vi "Read Array of the pixel to zone correspondences.vi"(8 "error in (no error)":errorcluster, 11 "Data in":refnum<class "Data.lvclass">) -> (0 "error out":errorcluster, 2 "Pixel <> Zone":T1, 3 "Data out":refnum<class "Data.lvclass">)   [LabVIEW 2018, in "Data.lvclass"]
uses:
  Data.lvclass
  SubVi's/Controls/CTL_Pixel_to_Zone_array.ctl
  Data.lvclass/Data.ctl
  Common_Resources.lvlib
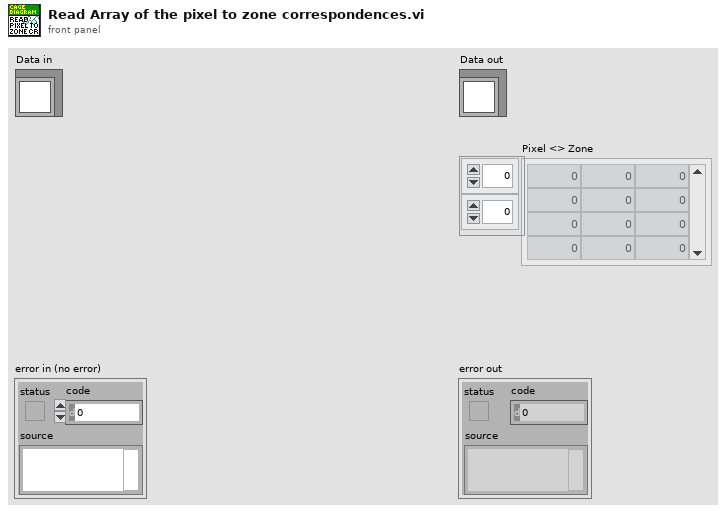
[diagram p1: front panel]
types:
  T1 = typedef "Common_Resources.lvlib/CTL_Pixel_to_Zone_array.ctl" = i8[][]
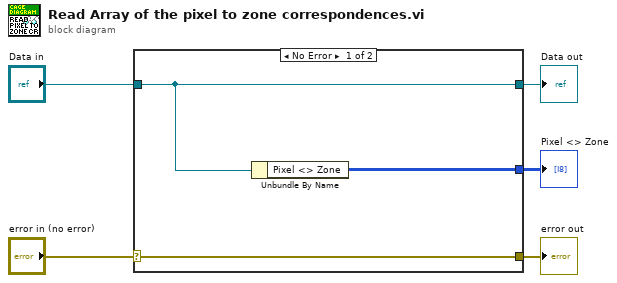
[diagram p0: block diagram]
diagram:
  n1 = case shown="No Error" "error in (no error)" {
    selector: "error in (no error)" -> [w8 w9]
    tunnel: [w8 w9] -> w4
    tunnel: [w7 w10] -> w2
    tunnel: "Data in" -> [w7 w10]
    tunnel: [w6 _] -> w1
    frame No Error {
      n2 = Unbundle By Name(w7) -> ("Pixel <> Zone"=w6:T1)
    }
    frame Error {
    }
  }
  "error out" <- w4
  "Data out" <- w2
  "Pixel <> Zone" <- w1
